vi "HL_R-1.vi"() -> ()   [LabVIEW 2015]
uses:
  <vilib>/MakerHub/LINX/Public/Peripherals/Digital/Digital Write N Chans.vi
  <vilib>/MakerHub/LINX/Public/Peripherals/Analog/Analog Read 1 Chan.vi
  <vilib>/MakerHub/LINX/Private/Local IO/LinxDigitalWrite.vi
  <vilib>/MakerHub/LINX/Public/Utilities/Check Channel.vi
  <vilib>/MakerHub/LINX/Public/Peripherals/Analog/Analog Read N Chans.vi
  <vilib>/MakerHub/LINX/Private/Local IO/LinxAnalogRead.vi
  <vilib>/MakerHub/LINX/Public/Utilities/Open Serial.vi
  <vilib>/MakerHub/LINX/Private/Utilties/Generate Error.vi
  <vilib>/MakerHub/LINX/LMH-LINX.lvlib
panel:
  in  "time post":u32
  in  "number of pulses":i32
  in  "low R - 1":dbl
  in  "peak delay":dbl
  out "Ref":dbl(graph)
  in  "LED":refnum<visa-resource-name>="N/A"
  out "3":dbl(graph)
  out "2":dbl(graph)
  out "4":dbl(graph)
  out "1":dbl(graph)
  out "pos":dbl
  in  "milliseconds to wait":u32
  in  "time pre":u32
  in  "Serial Port Analog":refnum<visa-resource-name>="N/A"
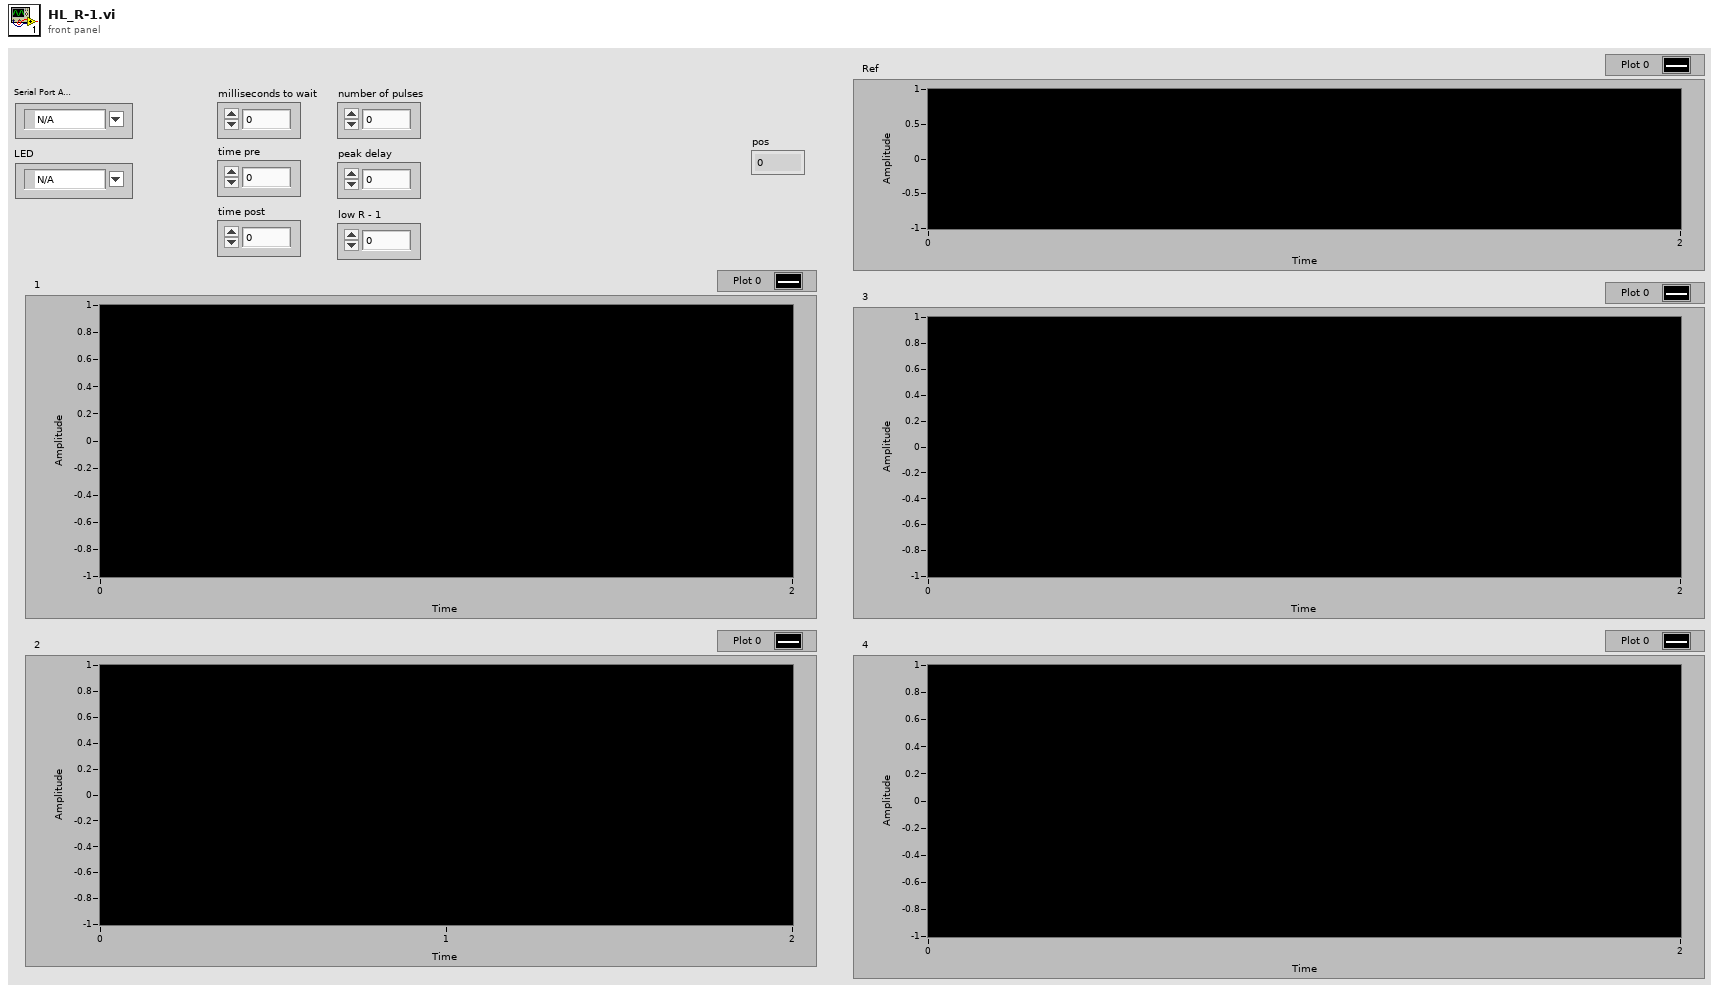
[diagram p1: front panel]
types:
  T1 = typedef "LMH-LINX.lvlib/LINX Ref.ctl" = cluster{"IO":T2, "Interface":T3, "LINX Device Config":T4}
  T2 = typedef "LMH-LINX.lvlib/Platform.ctl" = enum16{"Remote", "Local"}
  T3 = typedef "LMH-LINX.lvlib/Interface.ctl" = enum16{"Serial", "TCP"}
  T4 = typedef "LMH-LINX.lvlib/Device.lvlib/LINX Device Config.ctl" = cluster{"Interface":T3, "COM Port":refnum<visa-resource-name>, "TCP Configuration":T5, "Device Family":u8, "Device ID":u8, "Device Name":string, "TCP Ref":refnum<k5>, "Channels":T6}
  T5 = typedef "LMH-LINX.lvlib/Device.lvlib/TCP Config.ctl" = cluster{"IP Address":string, "Port":u16}
  T6 = typedef "LMH-LINX.lvlib/Channels.ctl" = cluster{"DI":u8[], "DO":u8[], "AI":u8[], "AO":u8[], "PWM":u8[], "QE":u8[], "UART":u8[], "I2C 2":u8[], "SPI":u8[], "CAN":u8[], "Servo":u8[], "AI Ref (V)":dbl, "AI Resolution (Bits)":u8, "AO Ref (V)":dbl, "AO Resolution (Bits)":u8}
  T7 = enum16{"open", "replace", "create", "open or create", "replace or create", "replace or create with confirmation"}
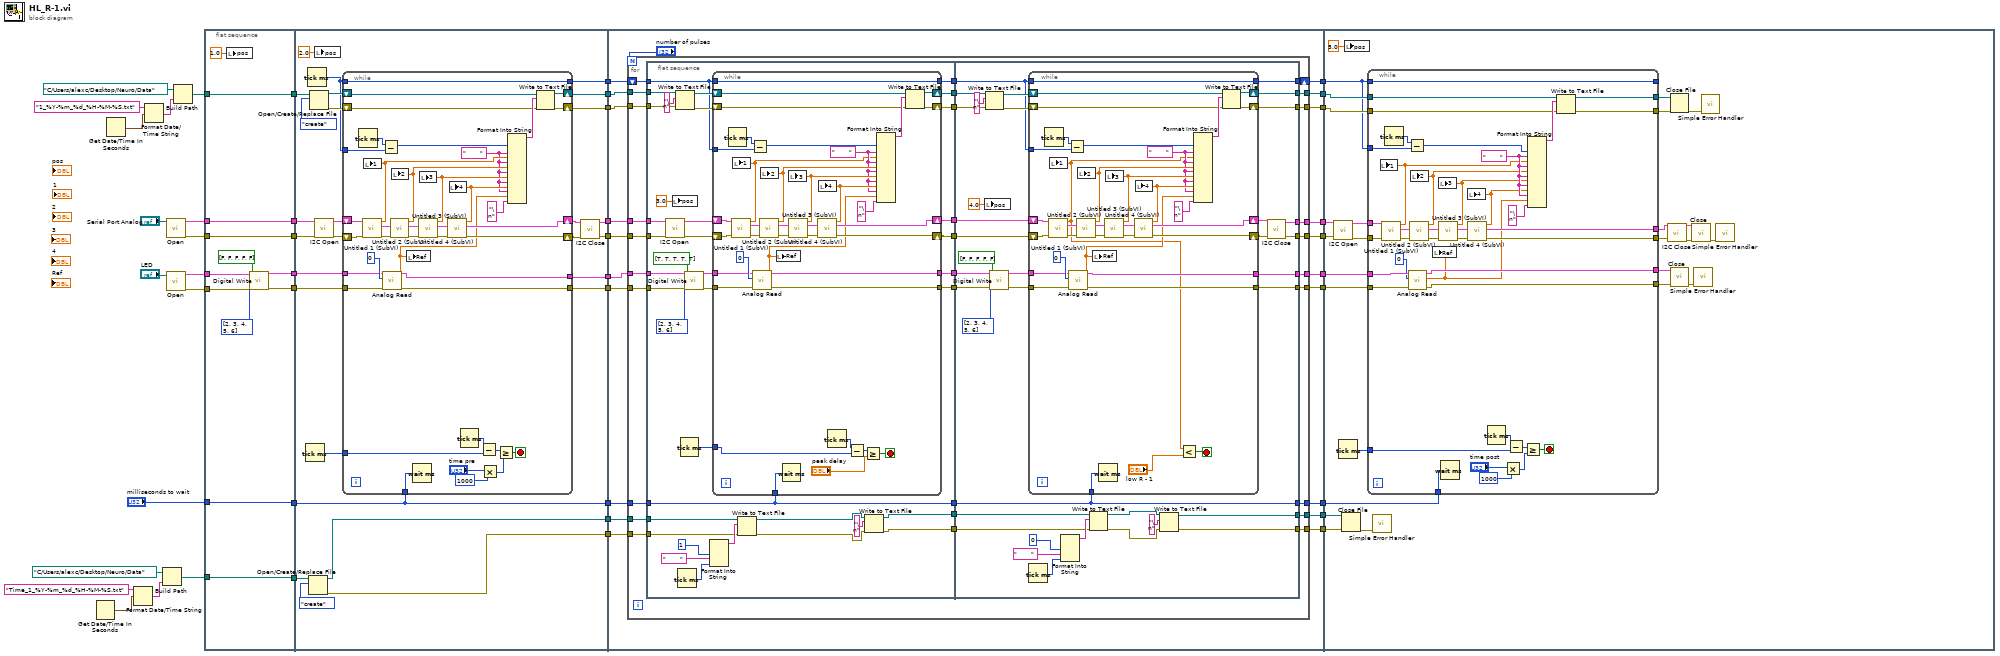
[diagram p0: block diagram]
diagram:
  n1 = Get Date/Time In Seconds() -> (seconds since 1Jan1904=w8:timestamp)
  n2 = Get Date/Time In Seconds() -> (seconds since 1Jan1904=w22:timestamp)
  n3 = Format Date/Time String(time format string (%c)="Time_1_%Y-%m_%d_%H-%M-%S.txt", seconds (now)=w8) -> (date/time string=w10:string)  [unwired: 1 in]
  n4 = Format Date/Time String(time format string (%c)="1_%Y-%m_%d_%H-%M-%S.txt", seconds (now)=w22) -> (date/time string=w24:string)  [unwired: 1 in]
  n5 = Build Path(base path=path "C:/Users/alexc/Desktop/Neuro/Data", name or relative path=w10) -> (appended path=w6:path)
  n6 = call-poly <vilib>:"Open.vi"("Serial Port"="Serial Port Analog") -> ("Error Out"=w28:errorcluster, "LINX Resource"=w29:T1)  [unwired: 8 in, 1 out]
  n7 = call-poly <vilib>:"Open.vi"("Serial Port"="LED") -> ("Error Out"=w19:errorcluster, "LINX Resource"=w20:T1)  [unwired: 8 in, 1 out]
  n8 = Build Path(base path=path "C:/Users/alexc/Desktop/Neuro/Data", name or relative path=w24) -> (appended path=w21:path)
  n9 = flat-sequence {
    tunnel: [w53] -> w44
    tunnel: [w52] -> w43
    tunnel: [w51] -> w40
    tunnel: [w46] -> w31
    tunnel: w29 -> [w53]
    tunnel: w28 -> [w52]
    tunnel: w21 -> [w51]
    tunnel: w20 -> [w50]
    tunnel: w19 -> [w49]
    tunnel: [w48] -> w18
    tunnel: [w47] -> w17
    tunnel: "milliseconds to wait" -> [w46]
    tunnel: [w45] -> w7
    tunnel: w6 -> [w45]
    tunnel: w44 -> [w83]
    tunnel: w43 -> [w82]
    tunnel: [w81] -> w42
    tunnel: [w80] -> w41
    tunnel: w40 -> [w79]
    tunnel: [w75] -> w39
    tunnel: [w74] -> w38
    tunnel: [w72] -> w37
    tunnel: w31 -> [w70]
    tunnel: [w70] -> w30
    tunnel: w18 -> [w64]
    tunnel: w17 -> [w63]
    tunnel: [w62] -> w16
    tunnel: w7 -> [w60]
    tunnel: [w59] -> w5
    tunnel: [w58] -> w4
    tunnel: [w57] -> w1
    tunnel: [w132] -> w36
    tunnel: [w131] -> w35
    tunnel: [w135] -> w34
    tunnel: [w134] -> w33
    tunnel: [w133] -> w32
    tunnel: w30 -> [w136]
    tunnel: w37 -> [w140]
    tunnel: w38 -> [w141]
    tunnel: w39 -> [w142]
    tunnel: w41 -> [w138]
    tunnel: w42 -> [w139]
    tunnel: w16 -> [w143]
    tunnel: [w130] -> w14
    tunnel: [w129] -> w13
    tunnel: [w128] -> w12
    tunnel: w5 -> [w127]
    tunnel: w4 -> [w126]
    tunnel: [w125] -> w3
    tunnel: [w124] -> w2
    tunnel: w1 -> [w123]
    tunnel: w32 -> [w334]
    tunnel: w33 -> [w335]
    tunnel: w34 -> [w321]
    tunnel: w35 -> [w339]
    tunnel: w36 -> [w343]
    tunnel: w14 -> [w338]
    tunnel: w13 -> [w325]
    tunnel: w12 -> [w324]
    tunnel: w3 -> [w319]
    tunnel: w2 -> [w318]
    frame #0 {
      n10 = local write "pos"(1.0 ("pos")) -> ()
      n11 = call-poly <vilib>:"Digital Write.vi"("Error In"=w49, "Values"=bool[] [FALSE, FALSE, FALSE, FALSE, FALSE], "DO Channels"=u8[] [2, 3, 4, 5, 6], "LINX Resource"=w50) -> ("Error Out"=w47:errorcluster, "LINX Resource"=w48:T1)  [unwired: 6 in]
    }
    frame #1 {
      n12 = Tick Count (ms)() -> (millisecond timer value=w71:u32)
      n13 = Tick Count (ms)() -> (millisecond timer value=w73:u32)
      n14 = Open/Create/Replace File(file path (use dialog)=w60, operation (0:open)=T7."create") -> (refnum out=w59:refnum<file>, error out=w58:errorcluster)  [unwired: 4 in, 1 out]
      n15 = Open/Create/Replace File(file path (use dialog)=w79, operation (0:open)=T7."create") -> (refnum out=w77:refnum<file>, error out=w76:errorcluster)  [unwired: 4 in, 1 out]
      n16 = local write "pos"(2.0 ("pos")) -> ()
      n17 = call <vilib>:"I2C Open.vi"("Error In"=w82, "LINX Resource"=w83) -> ("Error Out"=w68:errorcluster, "LINX Resource"=w69:T1)  [unwired: 8 in]
      n18 = while {
        tunnel: w73 -> [w115]
        shift-right: [w111] -> w75
        shift-left: w77 -> [w113]
        shift-right: [w110] -> w74
        shift-left: w76 -> [w112]
        tunnel: [w109] -> w72
        tunnel: w73 -> [w109]
        tunnel: w71 -> [w89]
        tunnel: w70 -> [w93]
        shift-right: [w106] -> w67
        shift-left: w69 -> [w108]
        shift-right: [w105] -> w66
        shift-left: w68 -> [w107]
        tunnel: w64 -> [w95]
        tunnel: w63 -> [w94]
        tunnel: [w92] -> w62
        tunnel: [w84] -> w57
        stop <- w88 stop-if-true
        w99 = "       "
        n19 = Tick Count (ms)() -> (millisecond timer value=w116:u32)
        n20 = call "Untitled 1 (SubVI).vi"("error in (no error)"=w107, "LINX Resource in"=w108) -> ("error out"=w121:errorcluster, "LINX Resource out"=w122:T1, "Numeric"=w103:dbl)  [unwired: 7 in]
        n21 = local write "1"(w103) -> ()
        n22 = Subtract(x=w116, y=w115) -> (x-y=w100:u32)
        n23 = call-poly <vilib>:"Analog Read.vi"("Error In"=w94, "Analog Channel"=u8 0, "LINX Resource"=w95) -> ("Error Out"=w84:errorcluster, "Voltage"=w96:dbl, "LINX Resource"=w92:T1)  [unwired: 5 in, 1 out]
        n24 = call "Untitled 2 (SubVI).vi"("error in (no error)"=w121, "LINX Resource in"=w122) -> ("error out"=w120:errorcluster, "LINX Resource"=w119:T1, "Numeric"=w102:dbl)  [unwired: 7 in]
        n25 = local write "2"(w102) -> ()
        n26 = local write "Ref"(w96) -> ()
        n27 = Wait (ms)(milliseconds to wait=w93) -> ()  [unwired: 1 out]
        n28 = call "Untitled 3 (SubVI).vi"("error in (no error)"=w120, "LINX Resource in"=w119) -> ("error out"=w117:errorcluster, "LINX Resource out"=w118:T1, "Numeric"=w101:dbl)  [unwired: 7 in]
        n29 = local write "3"(w101) -> ()
        n30 = call "Untitled 4 (SubVI).vi"("error in (no error)"=w117, "LINX Resource in"=w118) -> ("error out"=w105:errorcluster, "LINX Resource"=w106:T1, "Numeric"=w104:dbl)  [unwired: 7 in]
        n31 = local write "4"(w104) -> ()
        n32 = Tick Count (ms)() -> (millisecond timer value=w90:u32)
        n33 = Subtract(x=w90, y=w89) -> (x-y=w91:u32)
        n34 = Multiply(x="time pre", y=u32 1000) -> (x*y=w87:u32)
        n35 = Greater Or Equal?(x=w91, y=w87) -> (x >= y?=w88:bool)
        n36 = Format Into String(w100, w99, w103, w99, w102, w99, w101, w99, w104, w99, w96, "\n") -> (resulting string=w114:string)  [unwired: 3 in, 1 out]
        n37 = Write to Text File(file (use dialog)=w113, text=w114, error in=w112) -> (refnum out=w111:refnum<file>, error out=w110:errorcluster)  [unwired: 1 in, 1 out]
      }
      n38 = call <vilib>:"I2C Close.vi"("Error In"=w66, "LINX Resource"=w67) -> ("Error Out"=w80:errorcluster, "LINX Resource"=w81:T1)  [unwired: 8 in]
    }
    frame #2 {
      n39 = for {
        N: "number of pulses" -> [_]
        tunnel: w143 -> [w173]
        tunnel: w142 -> [w172]
        tunnel: w141 -> [w171]
        shift-right: [w158] -> w135
        shift-left: w140 -> [w168]
        tunnel: w139 -> [w170]
        tunnel: w138 -> [w169]
        tunnel: w136 -> [w160]
        tunnel: [w157] -> w134
        tunnel: [w156] -> w133
        tunnel: [w155] -> w132
        tunnel: [w154] -> w131
        tunnel: [w153] -> w130
        tunnel: [w152] -> w129
        tunnel: [w151] -> w128
        tunnel: w127 -> [w150]
        tunnel: w126 -> [w149]
        tunnel: [w146] -> w125
        tunnel: [w145] -> w124
        tunnel: w123 -> [w144]
        n40 = flat-sequence {
          tunnel: w173 -> [w205]
          tunnel: w172 -> [w202]
          tunnel: w171 -> [w201]
          tunnel: w170 -> [w194]
          tunnel: w169 -> [w193]
          tunnel: w168 -> [w190]
          tunnel: [w209] -> w167
          tunnel: [w208] -> w166
          tunnel: [w204] -> w165
          tunnel: [w203] -> w164
          tunnel: [w198] -> w163
          tunnel: [w197] -> w162
          tunnel: [w189] -> w161
          tunnel: w160 -> [w187]
          tunnel: [w187] -> w159
          tunnel: w150 -> [w185]
          tunnel: w149 -> [w184]
          tunnel: [w177] -> w148
          tunnel: [w176] -> w147
          tunnel: w144 -> [w174]
          tunnel: w167 -> [w276]
          tunnel: w166 -> [w275]
          tunnel: w165 -> [w270]
          tunnel: w164 -> [w269]
          tunnel: w163 -> [w272]
          tunnel: w162 -> [w271]
          tunnel: w161 -> [w268]
          tunnel: w159 -> [w261]
          tunnel: [w266] -> w158
          tunnel: [w265] -> w157
          tunnel: [w264] -> w156
          tunnel: [w263] -> w155
          tunnel: [w262] -> w154
          tunnel: [w261] -> w153
          tunnel: [w260] -> w152
          tunnel: [w259] -> w151
          tunnel: w148 -> [w254]
          tunnel: w147 -> [w253]
          tunnel: [w249] -> w146
          tunnel: [w248] -> w145
          frame #0 {
            n41 = call <vilib>:"I2C Open.vi"("Error In"=w193, "LINX Resource"=w194) -> ("Error Out"=w191:errorcluster, "LINX Resource"=w192:T1)  [unwired: 8 in]
            n42 = local write "pos"(3.0 ("pos")) -> ()
            n43 = Write to Text File(file (use dialog)=w202, text="\n", error in=w201) -> (refnum out=w200:refnum<file>, error out=w199:errorcluster)  [unwired: 1 in, 1 out]
            n44 = Tick Count (ms)() -> (millisecond timer value=w181:u32)
            n45 = Tick Count (ms)() -> (millisecond timer value=w175:u32)
            n46 = call-poly <vilib>:"Digital Write.vi"("Error In"=w174, "Values"=bool[] [TRUE, TRUE, TRUE, TRUE, TRUE], "DO Channels"=u8[] [2, 3, 4, 5, 6], "LINX Resource"=w205) -> ("Error Out"=w196:errorcluster, "LINX Resource"=w195:T1)  [unwired: 6 in]
            n47 = Format Into String(u32 1 ("input 1"), "       ", w181) -> (resulting string=w186:string)  [unwired: 3 in, 1 out]
            n48 = while {
              tunnel: w190 -> [w240]
              shift-right: [w236] -> w204
              shift-left: w200 -> [w238]
              shift-right: [w235] -> w203
              shift-left: w199 -> [w237]
              tunnel: [w234] -> w189
              tunnel: w190 -> [w234]
              tunnel: w187 -> [w219]
              shift-right: [w231] -> w209
              shift-left: w192 -> [w233]
              shift-right: [w230] -> w208
              shift-left: w191 -> [w232]
              tunnel: w195 -> [w221]
              tunnel: w196 -> [w220]
              tunnel: [w218] -> w198
              tunnel: [w217] -> w197
              tunnel: w175 -> [w211]
              stop <- w213 stop-if-true
              w225 = "       "
              n49 = Tick Count (ms)() -> (millisecond timer value=w241:u32)
              n50 = call "Untitled 1 (SubVI).vi"("error in (no error)"=w232, "LINX Resource in"=w233) -> ("error out"=w246:errorcluster, "LINX Resource out"=w247:T1, "Numeric"=w216:dbl)  [unwired: 7 in]
              n51 = local write "1"(w216) -> ()
              n52 = Subtract(x=w241, y=w240) -> (x-y=w226:u32)
              n53 = call-poly <vilib>:"Analog Read.vi"("Error In"=w220, "Analog Channel"=u8 0, "LINX Resource"=w221) -> ("Error Out"=w217:errorcluster, "Voltage"=w222:dbl, "LINX Resource"=w218:T1)  [unwired: 5 in, 1 out]
              n54 = call "Untitled 2 (SubVI).vi"("error in (no error)"=w246, "LINX Resource in"=w247) -> ("error out"=w245:errorcluster, "LINX Resource"=w244:T1, "Numeric"=w228:dbl)  [unwired: 7 in]
              n55 = local write "2"(w228) -> ()
              n56 = local write "Ref"(w222) -> ()
              n57 = Wait (ms)(milliseconds to wait=w219) -> ()  [unwired: 1 out]
              n58 = call "Untitled 3 (SubVI).vi"("error in (no error)"=w245, "LINX Resource in"=w244) -> ("error out"=w242:errorcluster, "LINX Resource out"=w243:T1, "Numeric"=w227:dbl)  [unwired: 7 in]
              n59 = local write "3"(w227) -> ()
              n60 = call "Untitled 4 (SubVI).vi"("error in (no error)"=w242, "LINX Resource in"=w243) -> ("error out"=w230:errorcluster, "LINX Resource"=w231:T1, "Numeric"=w229:dbl)  [unwired: 7 in]
              n61 = local write "4"(w229) -> ()
              n62 = Tick Count (ms)() -> (millisecond timer value=w214:u32)
              n63 = Subtract(x=w214, y=w211) -> (x-y=w215:u32)
              n64 = Greater Or Equal?(x=w215, y="peak delay") -> (x >= y?=w213:bool)
              n65 = Format Into String(w226, w225, w216, w225, w228, w225, w227, w225, w229, w225, w222, "\n") -> (resulting string=w239:string)  [unwired: 3 in, 1 out]
              n66 = Write to Text File(file (use dialog)=w238, text=w239, error in=w237) -> (refnum out=w236:refnum<file>, error out=w235:errorcluster)  [unwired: 1 in, 1 out]
            }
            n67 = Write to Text File(file (use dialog)=w185, text=w186, error in=w184) -> (refnum out=w179:refnum<file>, error out=w178:errorcluster)  [unwired: 1 in, 1 out]
            n68 = Write to Text File(file (use dialog)=w179, text="\n", error in=w178) -> (refnum out=w177:refnum<file>, error out=w176:errorcluster)  [unwired: 1 in, 1 out]
          }
          frame #1 {
            n69 = local write "pos"(4.0 ("pos")) -> ()
            n70 = Write to Text File(file (use dialog)=w270, text="\n", error in=w269) -> (refnum out=w278:refnum<file>, error out=w279:errorcluster)  [unwired: 1 in, 1 out]
            n71 = call-poly <vilib>:"Digital Write.vi"("Error In"=w271, "Values"=bool[] [FALSE, FALSE, FALSE, FALSE, FALSE], "DO Channels"=u8[] [2, 3, 4, 5, 6], "LINX Resource"=w272) -> ("Error Out"=w283:errorcluster, "LINX Resource"=w282:T1)  [unwired: 6 in]
            n72 = while {
              tunnel: w268 -> [w310]
              shift-right: [w306] -> w265
              shift-left: w278 -> [w308]
              shift-right: [w305] -> w264
              shift-left: w279 -> [w307]
              tunnel: [w304] -> w266
              tunnel: w268 -> [w304]
              tunnel: w261 -> [w289]
              shift-right: [w301] -> w274
              shift-left: w276 -> [w303]
              shift-right: [w300] -> w273
              shift-left: w275 -> [w302]
              tunnel: w282 -> [w291]
              tunnel: w283 -> [w290]
              tunnel: [w288] -> w260
              tunnel: [w287] -> w259
              stop <- w286 stop-if-true
              w295 = "       "
              n73 = Tick Count (ms)() -> (millisecond timer value=w311:u32)
              n74 = call "Untitled 1 (SubVI).vi"("error in (no error)"=w302, "LINX Resource in"=w303) -> ("error out"=w316:errorcluster, "LINX Resource out"=w317:T1, "Numeric"=w284:dbl)  [unwired: 7 in]
              n75 = local write "1"(w284) -> ()
              n76 = Subtract(x=w311, y=w310) -> (x-y=w296:u32)
              n77 = call-poly <vilib>:"Analog Read.vi"("Error In"=w290, "Analog Channel"=u8 0, "LINX Resource"=w291) -> ("Error Out"=w287:errorcluster, "Voltage"=w292:dbl, "LINX Resource"=w288:T1)  [unwired: 5 in, 1 out]
              n78 = call "Untitled 2 (SubVI).vi"("error in (no error)"=w316, "LINX Resource in"=w317) -> ("error out"=w315:errorcluster, "LINX Resource"=w314:T1, "Numeric"=w298:dbl)  [unwired: 7 in]
              n79 = local write "2"(w298) -> ()
              n80 = local write "Ref"(w292) -> ()
              n81 = Wait (ms)(milliseconds to wait=w289) -> ()  [unwired: 1 out]
              n82 = call "Untitled 3 (SubVI).vi"("error in (no error)"=w315, "LINX Resource in"=w314) -> ("error out"=w312:errorcluster, "LINX Resource out"=w313:T1, "Numeric"=w297:dbl)  [unwired: 7 in]
              n83 = local write "3"(w297) -> ()
              n84 = call "Untitled 4 (SubVI).vi"("error in (no error)"=w312, "LINX Resource in"=w313) -> ("error out"=w300:errorcluster, "LINX Resource"=w301:T1, "Numeric"=w299:dbl)  [unwired: 7 in]
              n85 = local write "4"(w299) -> ()
              n86 = Less?(x=w284, y="low R - 1") -> (x < y?=w286:bool)
              n87 = Format Into String(w296, w295, w284, w295, w298, w295, w297, w295, w299, w295, w292, "\n") -> (resulting string=w309:string)  [unwired: 3 in, 1 out]
              n88 = Write to Text File(file (use dialog)=w308, text=w309, error in=w307) -> (refnum out=w306:refnum<file>, error out=w305:errorcluster)  [unwired: 1 in, 1 out]
            }
            n89 = Tick Count (ms)() -> (millisecond timer value=w255:u32)
            n90 = Format Into String(u32 0 ("input 1"), "       ", w255) -> (resulting string=w258:string)  [unwired: 3 in, 1 out]
            n91 = Write to Text File(file (use dialog)=w254, text=w258, error in=w253) -> (refnum out=w251:refnum<file>, error out=w250:errorcluster)  [unwired: 1 in, 1 out]
            n92 = Write to Text File(file (use dialog)=w251, text="\n", error in=w250) -> (refnum out=w249:refnum<file>, error out=w248:errorcluster)  [unwired: 1 in, 1 out]
            n93 = call <vilib>:"I2C Close.vi"("Error In"=w273, "LINX Resource"=w274) -> ("Error Out"=w262:errorcluster, "LINX Resource"=w263:T1)  [unwired: 8 in]
          }
        }
      }
    }
    frame #3 {
      n94 = call <vilib>:"I2C Open.vi"("Error In"=w339, "LINX Resource"=w343) -> ("Error Out"=w336:errorcluster, "LINX Resource"=w337:T1)  [unwired: 8 in]
      n95 = Tick Count (ms)() -> (millisecond timer value=w333:u32)
      n96 = Close File(refnum=w319, error in=w318) -> (error out=w320:errorcluster)  [unwired: 1 out]
      n97 = local write "pos"(5.0 ("pos")) -> ()
      n98 = while {
        tunnel: w338 -> [w376]
        tunnel: w337 -> [w375]
        tunnel: w336 -> [w374]
        tunnel: [w368] -> _
        tunnel: w321 -> [w368]
        tunnel: w335 -> [w367]
        tunnel: w334 -> [w366]
        tunnel: w333 -> [w347]
        tunnel: [w365] -> w332
        tunnel: [w364] -> w331
        tunnel: [w363] -> w328
        tunnel: [w362] -> w327
        tunnel: w325 -> [w361]
        tunnel: w324 -> [w360]
        tunnel: [w359] -> w323
        tunnel: [w358] -> w322
        tunnel: w321 -> [w356]
        stop <- w348 stop-if-true
        w378 = "       "
        n99 = call "Untitled 1 (SubVI).vi"("error in (no error)"=w374, "LINX Resource in"=w375) -> ("error out"=w373:errorcluster, "LINX Resource out"=w382:T1, "Numeric"=w370:dbl)  [unwired: 7 in]
        n100 = local write "1"(w370) -> ()
        n101 = Tick Count (ms)() -> (millisecond timer value=w369:u32)
        n102 = Subtract(x=w369, y=w356) -> (x-y=w355:u32)
        n103 = call-poly <vilib>:"Analog Read.vi"("Error In"=w360, "Analog Channel"=u8 0, "LINX Resource"=w361) -> ("Error Out"=w358:errorcluster, "Voltage"=w354:dbl, "LINX Resource"=w359:T1)  [unwired: 5 in, 1 out]
        n104 = call "Untitled 2 (SubVI).vi"("error in (no error)"=w373, "LINX Resource in"=w382) -> ("error out"=w372:errorcluster, "LINX Resource"=w381:T1, "Numeric"=w353:dbl)  [unwired: 7 in]
        n105 = local write "2"(w353) -> ()
        n106 = local write "Ref"(w354) -> ()
        n107 = call "Untitled 3 (SubVI).vi"("error in (no error)"=w372, "LINX Resource in"=w381) -> ("error out"=w371:errorcluster, "LINX Resource out"=w380:T1, "Numeric"=w352:dbl)  [unwired: 7 in]
        n108 = local write "3"(w352) -> ()
        n109 = Wait (ms)(milliseconds to wait=w376) -> ()  [unwired: 1 out]
        n110 = call "Untitled 4 (SubVI).vi"("error in (no error)"=w371, "LINX Resource in"=w380) -> ("error out"=w362:errorcluster, "LINX Resource"=w363:T1, "Numeric"=w351:dbl)  [unwired: 7 in]
        n111 = local write "4"(w351) -> ()
        n112 = Tick Count (ms)() -> (millisecond timer value=w349:u32)
        n113 = Multiply(x="time post", y=u32 1000) -> (x*y=w346:u32)
        n114 = Subtract(x=w349, y=w347) -> (x-y=w350:u32)
        n115 = Greater Or Equal?(x=w350, y=w346) -> (x >= y?=w348:bool)
        n116 = Format Into String(w355, w378, w370, w378, w353, w378, w352, w378, w351, w378, w354, "\n") -> (resulting string=w379:string)  [unwired: 3 in, 1 out]
        n117 = Write to Text File(file (use dialog)=w367, text=w379, error in=w366) -> (refnum out=w365:refnum<file>, error out=w364:errorcluster)  [unwired: 1 in, 1 out]
      }
      n118 = call <vilib>:"Simple Error Handler.vi"("error in (no error)"=w320) -> ()  [unwired: 4 in, 5 out]
      n119 = call <vilib>:"I2C Close.vi"("Error In"=w327, "LINX Resource"=w328) -> ("Error Out"=w329:errorcluster, "LINX Resource"=w330:T1)  [unwired: 8 in]
      n120 = Close File(refnum=w332, error in=w331) -> (error out=w342:errorcluster)  [unwired: 1 out]
      n121 = call <vilib>:"Close.vi"("Error In"=w322, "LINX Resource"=w323) -> ("Error Out"=w326:errorcluster)  [unwired: 9 in]
      n122 = call <vilib>:"Close.vi"("Error In"=w329, "LINX Resource"=w330) -> ("Error Out"=w341:errorcluster)  [unwired: 9 in]
      n123 = call <vilib>:"Simple Error Handler.vi"("error in (no error)"=w326) -> ()  [unwired: 4 in, 5 out]
      n124 = call <vilib>:"Simple Error Handler.vi"("error in (no error)"=w342) -> ()  [unwired: 4 in, 5 out]
      n125 = call <vilib>:"Simple Error Handler.vi"("error in (no error)"=w341) -> ()  [unwired: 4 in, 5 out]
    }
  }
